vi "niScope Configure Trigger Immediate.vi"(0 "instrument handle":refnum<k15>, 11 "error in":errorcluster) -> (4 "instrument handle out":refnum<k15>, 15 "error out":errorcluster)   [LabVIEW 2020]
doc: "Configures common properties for immediate triggering. Immediate triggering means the digitizer triggers itself."
uses:
  niScope_32.dll
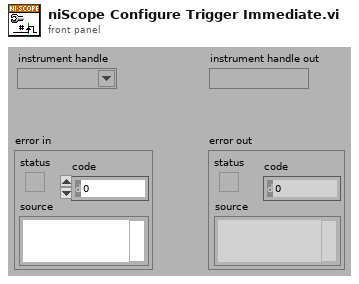
[diagram p1: front panel]
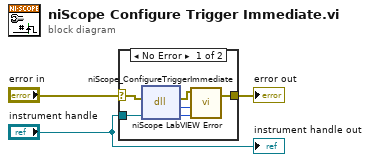
[diagram p0: block diagram]
diagram:
  n1 = case shown="No Error" "error in" {
    selector: "error in" -> [w5 w10]
    tunnel: [w6 w10] -> w2
    tunnel: "instrument handle" -> [w9 _]
    frame No Error {
      n2 = dll-call lib="niScope_*.*" fn="niScope_ConfigureTriggerImmediate"(error in=w5, "instrument handle"=w9) -> (error out=w4:errorcluster, "status"=w8:i32, "instrument handle"=w7:u32)  [unwired: 2 in, 1 out]
      n3 = call "niScope LabVIEW Error.vi"("instrument handle"=w7, "niScope error code (0)"=w8, "error in (no error)"=w4) -> ("error out"=w6:errorcluster)  [unwired: 2 in]
    }
    frame Error {
    }
  }
  "error out" <- w2
  "instrument handle out" <- "instrument handle"
